vi "ATSpectrograph_acceptCommand_enterControl.vi"(8 "error in (no error)":errorcluster, 11 "command_enterControl_Ctl":T1) -> (0 "error out":errorcluster, 2 "function return":i32, 3 "command_enterControl_Ctl out":T1)   [LabVIEW 2016, in "SALLV_ATSpectrograph.lvlib"]
doc: "int ATSpectrograph_shm_acceptCommand_enterControlLV(ATSpectrograph_command_enterControlLV *command_enterControl_Ctl );"
uses:
  SALLV_ATSpectrograph.lvlib
  DataTypes/command_enterControl.ctl
  SALLV_ATSpectrograph.so
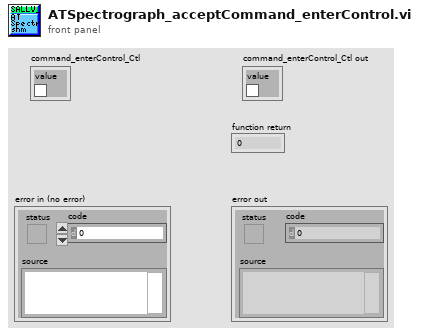
[diagram p1: front panel]
types:
  T1 = typedef "SALLV_ATSpectrograph.lvlib/command_enterControl.ctl" = cluster{"value":bool}
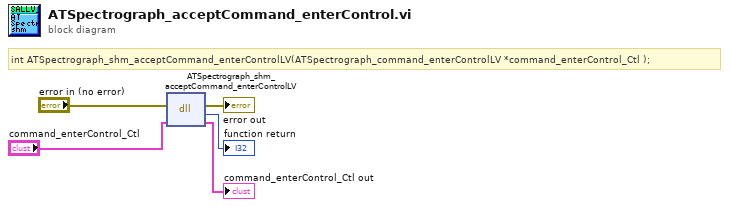
[diagram p0: block diagram]
diagram:
  # "int ATSpectrograph_shm_acceptCommand_enterControlLV(ATSpectrograph_command_enterControlLV *command_enterControl_Ctl );"
  n1 = dll-call lib="home/harini/tcs/SALLV_ATSpectrograph/SALLV_ATSpectrograph.*" fn="ATSpectrograph_shm_acceptCommand_enterControlLV"(error in="error in (no error)", "command_enterControl_Ctl"="command_enterControl_Ctl") -> (error out=→"error out":errorcluster, →"function return":i32, "command_enterControl_Ctl"=→"command_enterControl_Ctl out":T1)  [unwired: 2 in, 1 out]
